vi "LabvolutionSubmoduleCheck_Create_Delete_File.vi"(7 "Action":T1, 8 "error in (no error)":errorcluster) -> (0 "error out":errorcluster, 3 "Submodule Exists":bool)   [LabVIEW 2018]
uses:
  LabvolutionSubmoduleCheck_File_Action..enum.ctl
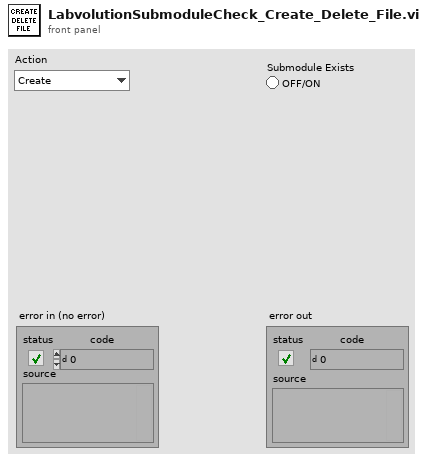
[diagram p1: front panel]
types:
  T1 = typedef "LabvolutionSubmoduleCheck_File_Action..enum.ctl" = enum16{"Create", "Remove", "Check"}
  T2 = enum16{"open", "replace", "create", "open or create", "replace or create", "replace or create with confirmation"}
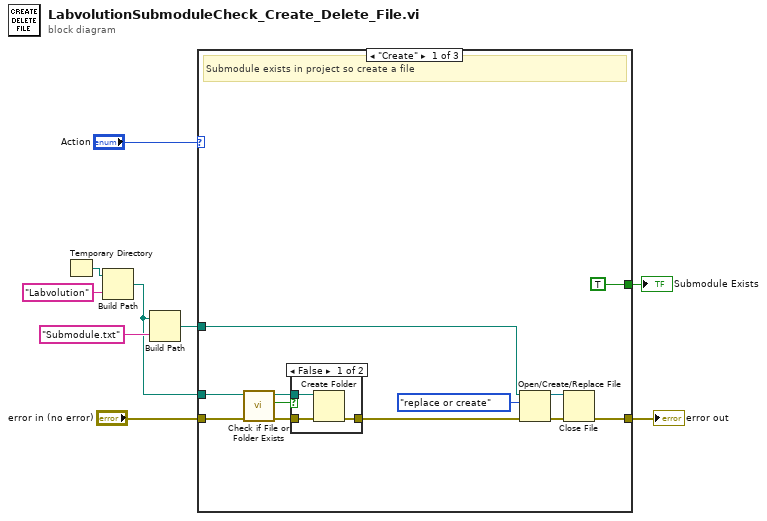
[diagram p0: block diagram]
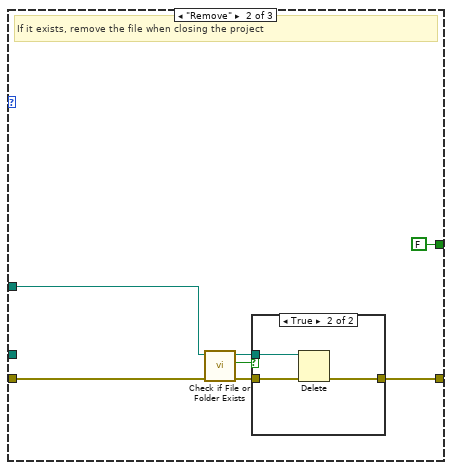
[diagram p3: hidden frame]
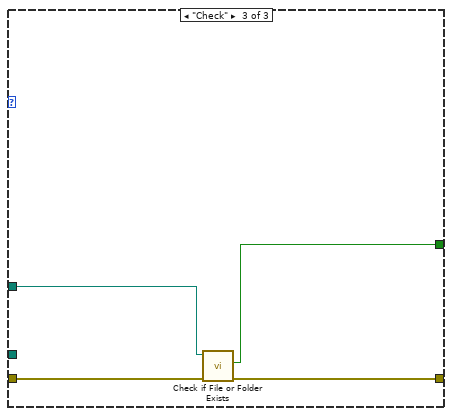
[diagram p5: hidden frame]
diagram:
  n1 = Temporary Directory() -> (w7:path)
  n2 = Build Path(base path=w7, name or relative path="Labvolution") -> (appended path=w2:path)
  n3 = Build Path(base path=w2, name or relative path="Submodule.txt") -> (appended path=w4:path)
  n4 = case shown="\"Create\"" "Action" {
    tunnel: "error in (no error)" -> [w12 w32 w40]
    tunnel: w4 -> [w21 w31 w39]
    tunnel: [w17 w27 w38] -> w3
    tunnel: w2 -> [w11 _ _]
    tunnel: [TRUE FALSE w37] -> w1
    frame "Create" {
      # "Submodule exists in project so create a file"
      n5 = call <vilib>:"Check if File or Folder Exists.vi"("error in (no error)"=w12, "path"=w11) -> ("error out"=w16:errorcluster, "file or folder exists?"=w14:bool, "dup path"=w15:path)  [unwired: 7 in]
      n6 = case shown="False" w14 {
        tunnel: w16 -> [w23 w25]
        tunnel: w15 -> [w24 _]
        tunnel: [w22 w25] -> w13
        frame False {
          n7 = Create Folder(path (use dialog)=w24, error in=w23) -> (error out=w22:errorcluster)  [unwired: 1 in, 2 out]
        }
        frame True {
        }
      }
      n8 = Open/Create/Replace File(file path (use dialog)=w21, error in=w13, operation (0:open)=T2."replace or create") -> (refnum out=w19:refnum<file>, error out=w18:errorcluster)  [unwired: 3 in, 1 out]
      n9 = Close File(refnum=w19, error in=w18) -> (error out=w17:errorcluster)  [unwired: 1 out]
    }
    frame "Remove" {
      # "If it exists, remove the file when closing the project"
      n10 = call <vilib>:"Check if File or Folder Exists.vi"("error in (no error)"=w32, "path"=w31) -> ("error out"=w30:errorcluster, "file or folder exists?"=w28:bool, "dup path"=w29:path)  [unwired: 7 in]
      n11 = case shown="True" w28 {
        tunnel: w30 -> [w33 w35]
        tunnel: w29 -> [_ w36]
        tunnel: [w33 w34] -> w27
        frame False {
        }
        frame True {
          n12 = Delete(path (use dialog)=w36, error in=w35) -> (error out=w34:errorcluster)  [unwired: 3 in, 2 out]
        }
      }
    }
    frame "Check" {
      n13 = call <vilib>:"Check if File or Folder Exists.vi"("error in (no error)"=w40, "path"=w39) -> ("error out"=w38:errorcluster, "file or folder exists?"=w37:bool)  [unwired: 7 in, 1 out]
    }
  }
  "error out" <- w3
  "Submodule Exists" <- w1
